vi "DSF.Engine.Interface.Set RT FIFO.vi"(8 "error in (no error)":errorcluster, 10 "RT FIFO":refnum<k33>, 11 "Interface in":refnum<class "DSF.Engine.Interface.lvclass">) -> (0 "error out":errorcluster, 3 "Interface out":refnum<class "DSF.Engine.Interface.lvclass">)   [LabVIEW 2016, in "DSF.Engine.lvlib" / "DSF.Engine.Interface.lvclass"]
uses:
  DSF.Engine.Interface.lvclass
  DSF.Engine.Interface.RT FIFO Data.ctl
  DSF.Engine.Interface.lvclass/DSF.Engine.Interface.ctl
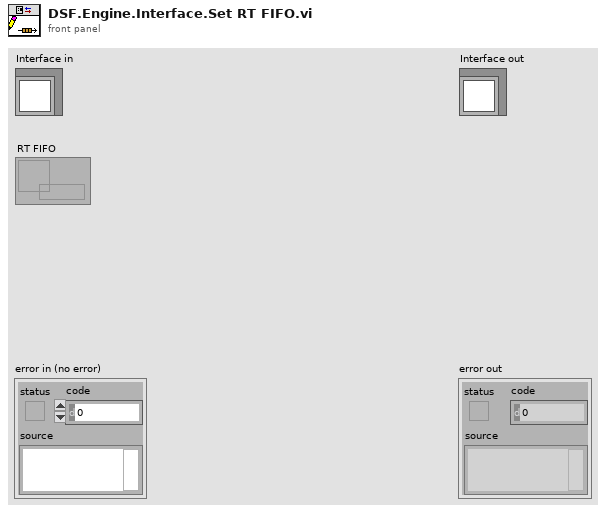
[diagram p1: front panel]
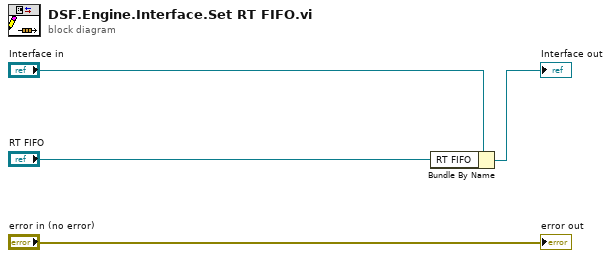
[diagram p0: block diagram]
diagram:
  n1 = Bundle By Name(cluster="Interface in", "RT FIFO"="RT FIFO") -> (→"Interface out":refnum<class "DSF.Engine.Interface.lvclass">)
  "error out" <- "error in (no error)"
